vi "SaveBrowerProject.vi"(8 "error in (no error)":errorcluster, 11 "BrowerController in":refnum<class "BrowerController.lvclass">) -> (0 "error out":errorcluster, 3 "BrowerController out":refnum<class "BrowerController.lvclass">)   [LabVIEW 2015, in "BrowerController.lvclass"]
uses:
  BrowerController.lvclass
  BrowerController.lvclass/BrowerController.ctl
  File IO/Controllers/Messages/SaveProject_Msg/SaveProject_Msg.lvclass/SaveProject_Msg.ctl
  <vilib>/ActorFramework/Message Enqueuer/Message Enqueuer.lvclass/Message Enqueuer.ctl
  <vilib>/ActorFramework/Message Enqueuer/Enqueue.vi
  <vilib>/ActorFramework/Message Priority Queue/Priority Enqueue.vi
  File IO/Controllers/Messages/SaveProject_Msg/SaveProject_Msg.lvclass
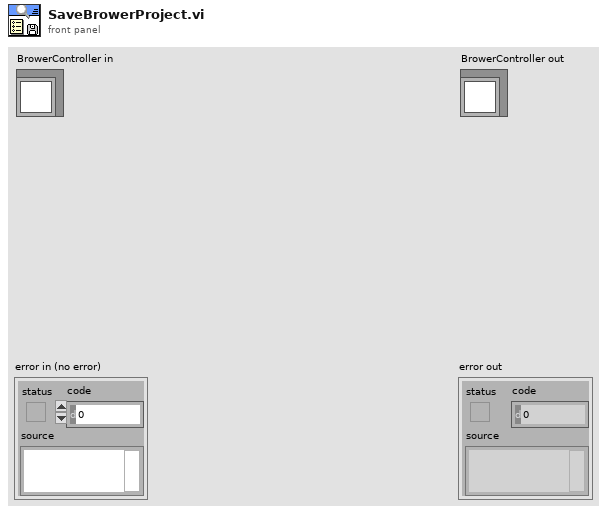
[diagram p1: front panel]
types:
  T1 = enum16{"open", "replace", "create", "open or create", "replace or create", "replace or create with confirmation"}
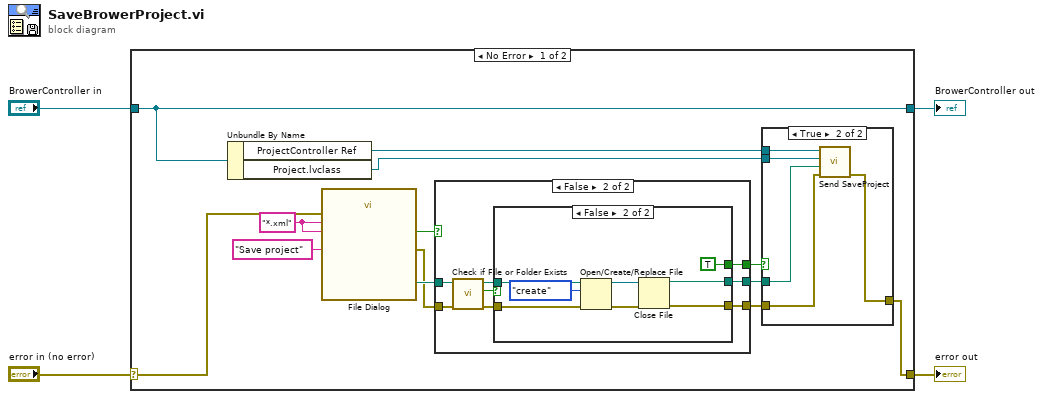
[diagram p0: block diagram]
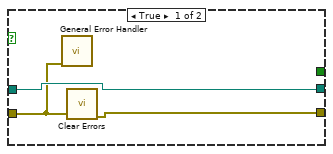
[diagram p2: hidden frame]
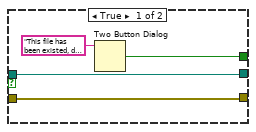
[diagram p3: hidden frame]
diagram:
  n1 = case shown="No Error" "error in (no error)" {
    selector: "error in (no error)" -> [w12 w48]
    tunnel: [w11 w48] -> w3
    tunnel: [w13 w47] -> w1
    tunnel: "BrowerController in" -> [w13 w47]
    frame No Error {
      w15 = "*.xml" ("pattern (all files)")
      n2 = Unbundle By Name(w13) -> ("ProjectController Ref"=w17:refnum<class "Message Enqueuer.lvclass">, "Project.lvclass"=w16:refnum<class "BrowerComponent.lvclass">)
      n3 = call "File Dialog"("prompt"="Save project", "error in"=w12, "pattern (all files)"=w15, "pattern label"=w15) -> ("selected path"=w10:path, "cancelled"=w6:bool, "error out"=w5:errorcluster)  [unwired: 8 in, 1 out]
      n4 = case shown="False" w6 {
        tunnel: w10 -> [w19 w28]
        tunnel: [w19 w24] -> w9
        tunnel: [w20 w23] -> w8
        tunnel: [_ w22] -> w7
        tunnel: w5 -> [w18 w21]
        frame True {
          n5 = call <vilib>:"General Error Handler.vi"("error in (no error)"=w18) -> ()  [unwired: 10 in, 5 out]
          n6 = call <vilib>:"Clear Errors.vi"("error in (no error)"=w18) -> ("error out"=w20:errorcluster)  [unwired: 5 in, 1 out]
        }
        frame False {
          n7 = call <vilib>:"Check if File or Folder Exists.vi"("error in (no error)"=w21, "path"=w28) -> ("error out"=w25:errorcluster, "file or folder exists?"=w27:bool, "dup path"=w26:path)  [unwired: 7 in]
          n8 = case shown="False" w27 {
            tunnel: w26 -> [w29 w40]
            tunnel: w25 -> [w30 w39]
            tunnel: [w30 w35] -> w23
            tunnel: [w29 w34] -> w24
            tunnel: [w31 TRUE ("T button?")] -> w22
            frame True {
              n9 = Two Button Dialog(message="This file has been existed, do you want to replace it!") -> (T button?=w31:bool)  [unwired: 2 in]
            }
            frame False {
              n10 = Open/Create/Replace File(file path (use dialog)=w40, error in=w39, operation (0:open)=T1."create") -> (refnum out=w37:refnum<file>, error out=w36:errorcluster)  [unwired: 3 in, 1 out]
              n11 = Close File(refnum=w37, error in=w36) -> (path=w34:path, error out=w35:errorcluster)
            }
          }
        }
      }
      n12 = case shown="True" w7 {
        tunnel: w17 -> [_ w46]
        tunnel: w16 -> [_ w45]
        tunnel: [w41 w44] -> w11
        tunnel: w9 -> [_ w43]
        tunnel: w8 -> [w41 w42]
        frame False {
        }
        frame True {
          n13 = call "Send SaveProject.vi"("error in (no error)"=w42, "Path"=w43, "BrowerComponent"=w45, "Message Enqueuer"=w46) -> ("error out"=w44:errorcluster)  [unwired: 6 in, 1 out]
        }
      }
    }
    frame Error {
    }
  }
  "error out" <- w3
  "BrowerController out" <- w1
